vi "Write commandFactory.vi"(10 "commandFactory":refnum<class "ICommandFactory.lvclass">, 11 "Model in":refnum<class "Model.lvclass">) -> (3 "Model out":refnum<class "Model.lvclass">)   [LabVIEW 2013, in "Model.lvclass"]
uses:
  Model.lvclass
  ICommandFactory/ICommandFactory.lvclass
  Model.lvclass/Model.ctl
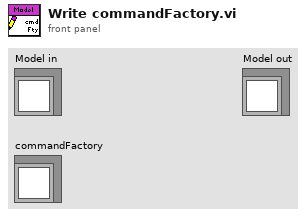
[diagram p1: front panel]
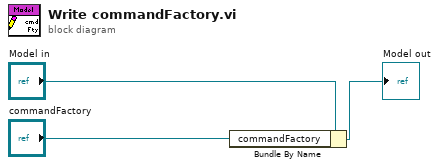
[diagram p0: block diagram]
diagram:
  n1 = Bundle By Name(cluster="Model in", "commandFactory"="commandFactory") -> (→"Model out":refnum<class "Model.lvclass">)
